vi "Pin Height Determination.vi"(8 "Error In":errorcluster, 10 "Pin number from Edge detection":enum16{"1", "2", "3", "4", "5"}(ring), 11 "Pixel Value of Pin from Highest Pixel Abscissa Determination VI":dbl) -> (0 "Error Out":errorcluster, 3 "Height in Pixels":dbl)   [LabVIEW 2016]
panel:
  in  "Pin 5 - Pixel Value of Pin Zero Reference":dbl=494.0 format="%#_13g"
  in  "Pin 4 - Pixel Value of Pin Zero Reference":dbl=360.0 format="%#_13g"
  in  "Pin 3 - Pixel Value of Pin Zero Reference":dbl=486.0 format="%#_13g"
  in  "Pin 2 - Pixel Value of Pin Zero Reference":dbl=352.0 format="%#_13g"
  in  "Pin 1 - Pixel Value of Pin Zero Reference":dbl=495.0
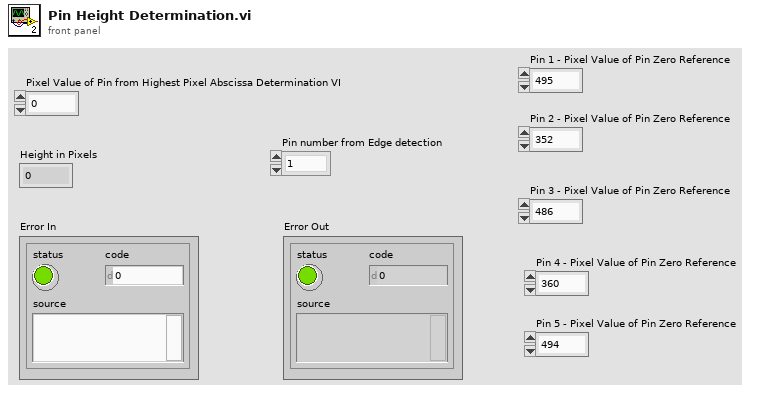
[diagram p1: front panel]
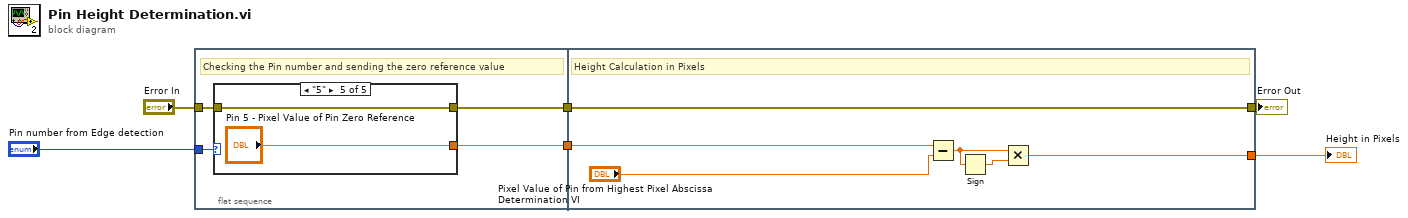
[diagram p0: block diagram]
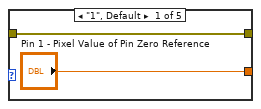
[diagram p2: hidden frame]
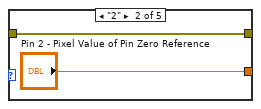
[diagram p3: hidden frame]
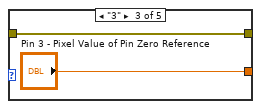
[diagram p4: hidden frame]
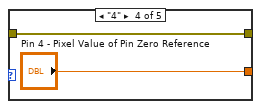
[diagram p5: hidden frame]
diagram:
  n1 = flat-sequence {
    tunnel: "Pin number from Edge detection" -> [w10]
    tunnel: "Error In" -> [w9]
    tunnel: [w8] -> w6
    tunnel: [w7] -> w5
    tunnel: w6 -> [w25]
    tunnel: [w25] -> w2
    tunnel: w5 -> [w24]
    tunnel: [w21] -> w1
    frame #0 {
      # "Checking the Pin number and sending the zero reference value"
      n2 = case shown="\"5\"" w10 {
        tunnel: w9 -> [w12 w13 w15 w17 w19]
        tunnel: [w12 w13 w15 w17 w19] -> w8
        tunnel: ["Pin 1 - Pixel Value of Pin Zero Reference" "Pin 2 - Pixel Value of Pin Zero Reference" "Pin 3 - Pixel Value of Pin Zero Reference" "Pin 4 - Pixel Value of Pin Zero Reference" "Pin 5 - Pixel Value of Pin Zero Reference"] -> w7
        frame "1", Default {
        }
        frame "2" {
        }
        frame "3" {
        }
        frame "4" {
        }
        frame "5" {
        }
      }
    }
    frame #1 {
      # "Height Calculation in Pixels"
      n3 = Subtract(x=w24, y="Pixel Value of Pin from Highest Pixel Abscissa Determination VI") -> (x-y=w22:dbl)
      n4 = Sign(1:w22) -> (0:w23:dbl)
      n5 = Multiply(x=w22, y=w23) -> (x*y=w21:dbl)
    }
  }
  "Error Out" <- w2
  "Height in Pixels" <- w1
